vi "ROI选择信息输出子VI.vi"(0 "Image In":T4, 1 "标注尺寸信息？":bool=TRUE, 5 "缺陷编号":u32, 7 "Current ROI Tool":u32(ring)=8 items=["Zoom Tool"=8, "Selection Tool"=0, "Pan Tool"=9, "Point Tool"=1, "Line Tool"=2, "Rectangle Tool"=3, "Rotated Rectangle Tool"=12, "Polyline Tool"=10, "Polygon Tool"=5, "Freehand Tool"=11, "Closed Freehand Tool"=6, "Ellipse Tool"=4, "Annulus Tool"=7], 9 "Color Palette":cluster{"Red":u8, "Green":u8, "Blue":u8}[](array[cluster]), 11 "X向分辨率（mm/p）":dbl, 12 "Y向分辨率（mm/p)":dbl) -> (2 "Cancelled":bool, 3 "ROI Descriptor":T1 {"Contours"."Type" items=["No Selection", "Point", "Line", "Rectangle", "Oval", "Polygon", "Freehand Region", "Annulus", "Unused2", "Unused3", "Broken Line", "Freehand Line", "Rotated Rectangle"]}, 4 "矩形缺陷尺寸信息":string, 6 "线性缺陷尺寸信息":string, 8 "矩形缺陷坐标":T2, 10 "线性缺陷坐标":T3 {"Start X" scale=0.0..1024.0; "End X" scale=0.0..1024.0}, 13 "矩形缺陷长":dbl format="%#_1g", 14 "矩形缺陷宽":dbl format="%#_1g", 15 "线性缺陷长度":dbl format="%#_1g")   [LabVIEW 2018]
uses:
  <vilib>/vision/Image Controls.llb/IMAQ Image.ctl
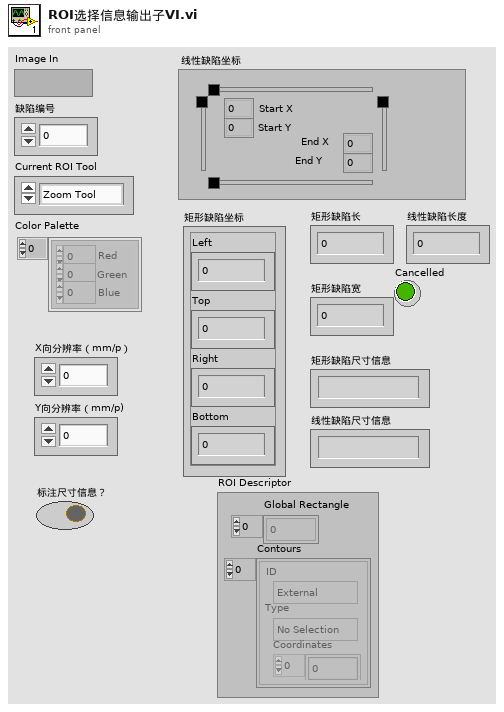
[diagram p1: front panel]
types:
  T1 = typedef "ROI Descriptor" = cluster{"Global Rectangle":i32[], "Contours":cluster{"ID":enum32{"External", "Internal"}, "Type":u32, "Coordinates":i32[]}[]}
  T2 = cluster{"Left":i32, "Top":i32, "Right":i32, "Bottom":i32}
  T3 = typedef "IMAQ Line" = cluster{"Start X":i32, "Start Y":i32, "End X":i32, "End Y":i32}
  T4 = typedef "IMAQ Image.ctl" = refnum<image>
  T5 = typedef "IMAQ Rectangle" = cluster{"Left":i32, "Top":i32, "Right":i32, "Bottom":i32, "Rotation":dbl}
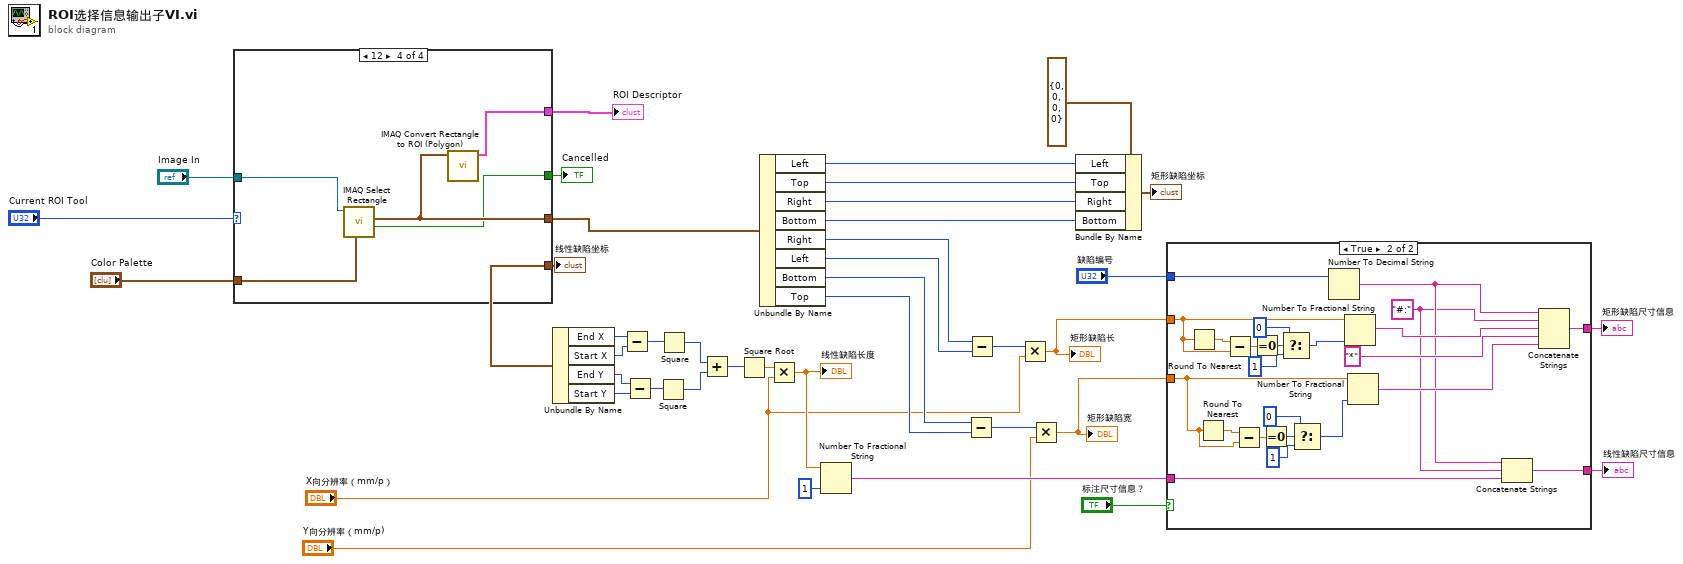
[diagram p0: block diagram]
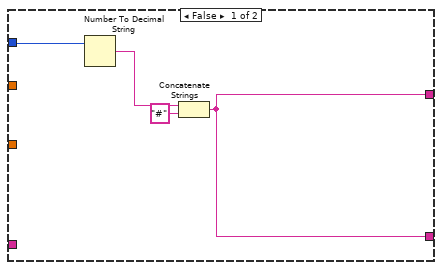
[diagram p2: hidden frame]
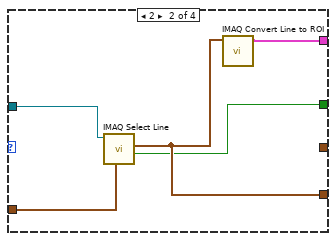
[diagram p4: hidden frame]
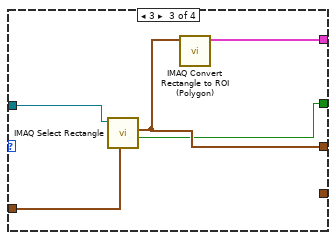
[diagram p5: hidden frame]
diagram:
  n1 = case shown="12" "Current ROI Tool" {
    tunnel: "Image In" -> [_ w45 w50 w55]
    tunnel: "Color Palette" -> [_ w44 w49 w54]
    tunnel: [_ _ w48 w53] -> w4
    tunnel: [_ w43 _ _] -> w29
    tunnel: [_ w42 w47 w52] -> w1
    tunnel: [_ w41 w46 w51] -> w2
    frame 0, Default {
    }
    frame 2 {
      n2 = call "IMAQ Select Line"("Color Palette"=w44, "Image In"=w45) -> ("Cancelled"=w41:bool, "Line"=w43:T3)  [unwired: 6 in, 2 out]
      n3 = call "IMAQ Convert Line to ROI"("Line"=w43) -> ("ROI Descriptor"=w42:T1)  [unwired: 8 in, 1 out]
    }
    frame 3 {
      n4 = call "IMAQ Select Rectangle"("Color Palette"=w49, "Image In"=w50) -> ("Cancelled"=w46:bool, "Rectangle"=w48:T5)  [unwired: 6 in, 2 out]
      n5 = call "IMAQ Convert Rectangle to ROI (Polygon)"("Rectangle"=w48) -> ("ROI Descriptor"=w47:T1)  [unwired: 7 in, 2 out]
    }
    frame 12 {
      n6 = call "IMAQ Select Rectangle"("Color Palette"=w54, "Image In"=w55) -> ("Cancelled"=w51:bool, "Rectangle"=w53:T5)  [unwired: 6 in, 2 out]
      n7 = call "IMAQ Convert Rectangle to ROI (Polygon)"("Rectangle"=w53) -> ("ROI Descriptor"=w52:T1)  [unwired: 7 in, 2 out]
    }
  }
  "线性缺陷坐标" <- w29
  "Cancelled" <- w2
  "ROI Descriptor" <- w1
  n8 = Unbundle By Name(w29) -> ("End X"=w28:i32, "Start X"=w27:i32, "End Y"=w24:i32, "Start Y"=w23:i32)
  n9 = Subtract(x=w28, y=w27) -> (x-y=w26:i32)
  n10 = Subtract(x=w24, y=w23) -> (x-y=w25:i32)
  n11 = Square(x=w25) -> (x^2=w21:i32)
  n12 = Square(x=w26) -> (x^2=w22:i32)
  n13 = Add(x=w22, y=w21) -> (x+y=w20:i32)
  n14 = Square Root(x=w20) -> (sqrt(x)=w12:dbl)
  n15 = Unbundle By Name(w4) -> ("Left"=w34:i32, "Top"=w32:i32, "Right"=w35:i32, "Bottom"=w33:i32, "Right"=w16:i32, "Left"=w15:i32, "Bottom"=w14:i32, "Top"=w13:i32)
  n16 = Multiply(x=w12, y="X向分辨率（mm/p）") -> (x*y=w9:dbl)
  "线性缺陷长度" <- w9
  n17 = Number To Fractional String(number=w9, precision (6)=i16 1 ("精度(6)")) -> (F-format string=w18:string)  [unwired: 2 in]
  n18 = Subtract(x=w14, y=w13) -> (x-y=w8:i32)
  n19 = Subtract(x=w16, y=w15) -> (x-y=w11:i32)
  n20 = Multiply(x=w11, y="X向分辨率（mm/p）") -> (x*y=w10:dbl)
  "矩形缺陷长" <- w10
  n21 = Multiply(x=w8, y="Y向分辨率（mm/p)") -> (x*y=w6:dbl)
  "矩形缺陷宽" <- w6
  n22 = Bundle By Name(cluster=T2 {"Left"=0, "Top"=0, "Right"=0, "Bottom"=0}, "Left"=w34, "Top"=w32, "Right"=w35, "Bottom"=w33) -> (→"矩形缺陷坐标":T2)
  n23 = case shown="True" "标注尺寸信息？" {
    tunnel: "缺陷编号" -> [w59 w79]
    tunnel: [w56 w78] -> w30
    tunnel: w18 -> [_ w75]
    tunnel: [w56 w74] -> w17
    tunnel: w10 -> [_ w68]
    tunnel: w6 -> [_ w71]
    frame False {
      n24 = Number To Decimal String(number=w59) -> (decimal integer string=w58:string)  [unwired: 1 in]
      n25 = Concatenate Strings(w58, "#" ("字符串")) -> (w56:string)
    }
    frame True {
      w76 = "#:" ("String")
      n26 = Round To Nearest(number=w68) -> (nearest integer value=w70:dbl)
      n27 = Round To Nearest(number=w71) -> (nearest integer value=w72:dbl)
      n28 = Subtract(x=w70, y=w68) -> (x-y=w69:dbl)
      n29 = Subtract(x=w72, y=w71) -> (x-y=w73:dbl)
      n30 = Equal To 0?(x=w69) -> (x = 0?=w63:bool)
      n31 = Equal To 0?(x=w73) -> (x = 0?=w67:bool)
      n32 = Select(t=i16 0, s=w63, f=i16 1 ("精度(6)")) -> (s? t:f=w60:i16)
      n33 = Select(t=i16 0, s=w67, f=i16 1 ("精度(6)")) -> (s? t:f=w64:i16)
      n34 = Number To Decimal String(number=w79) -> (decimal integer string=w77:string)  [unwired: 1 in]
      n35 = Number To Fractional String(number=w68, precision (6)=w60) -> (F-format string=w82:string)  [unwired: 2 in]
      n36 = Number To Fractional String(number=w71, precision (6)=w64) -> (F-format string=w80:string)  [unwired: 2 in]
      n37 = Concatenate Strings(w77, w76, w75) -> (w74:string)
      n38 = Concatenate Strings(w77, w76, w82, "*" ("String"), w80) -> (w78:string)
    }
  }
  "矩形缺陷尺寸信息" <- w30
  "线性缺陷尺寸信息" <- w17
